vi "FP behavior P-Wall.vi"(1 "Behavior\nVelocity":dbl=20.0, 2 "Activate?":bool=TRUE, 3 "IR Sensors":T1(array[cluster])) -> (0 "P-Wall Array":dbl[](array[numeric]))   [LabVIEW 2014]
doc: "This vi creates a array based upon the value of the PBow IR sensor reading."
uses:
  <vilib>/addons/control/pid/pid.llb/PID (DBL).vi
  <vilib>/addons/control/pid/NI_PID_pid.lvlib
panel:
  out "HPort Setpoint":dbl=40.0 format="%#_13g"
  out "Half-Port\nSensor":string
  out "Port Setpoint":dbl=40.0 format="%#_13g"
  out "steer":dbl format="%.2f"
  out "Port Side Sensor":string
  out "Waveform Graph":cluster{dbl, dbl, dbl[]}(graph)
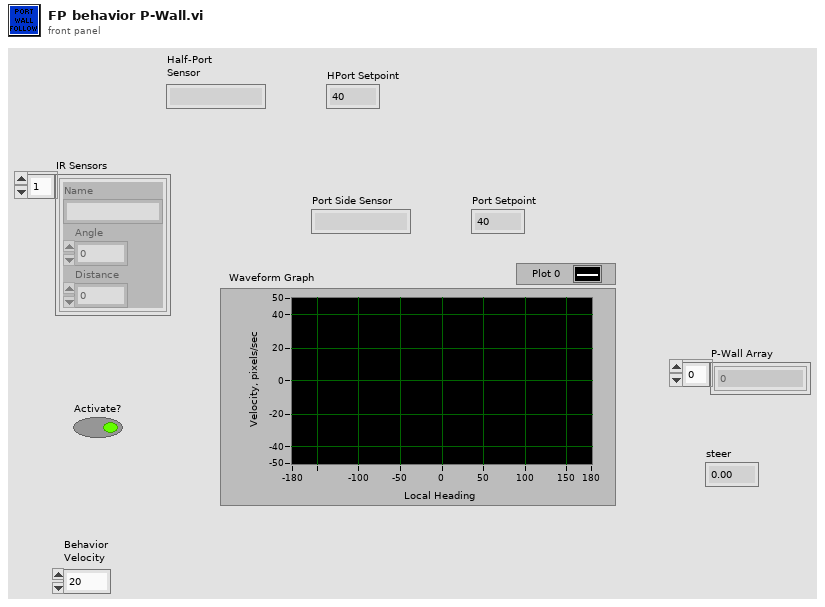
[diagram p1: front panel]
types:
  T1 = cluster{"Name":string, "Angle":dbl, "Distance":dbl}[]
  T2 = cluster{"proportional gain (Kc)":dbl, "integral time (Ti, min)":dbl, "derivative time (Td, min)":dbl}
  T3 = cluster{"Name":string, "Angle":dbl, "Distance":dbl}
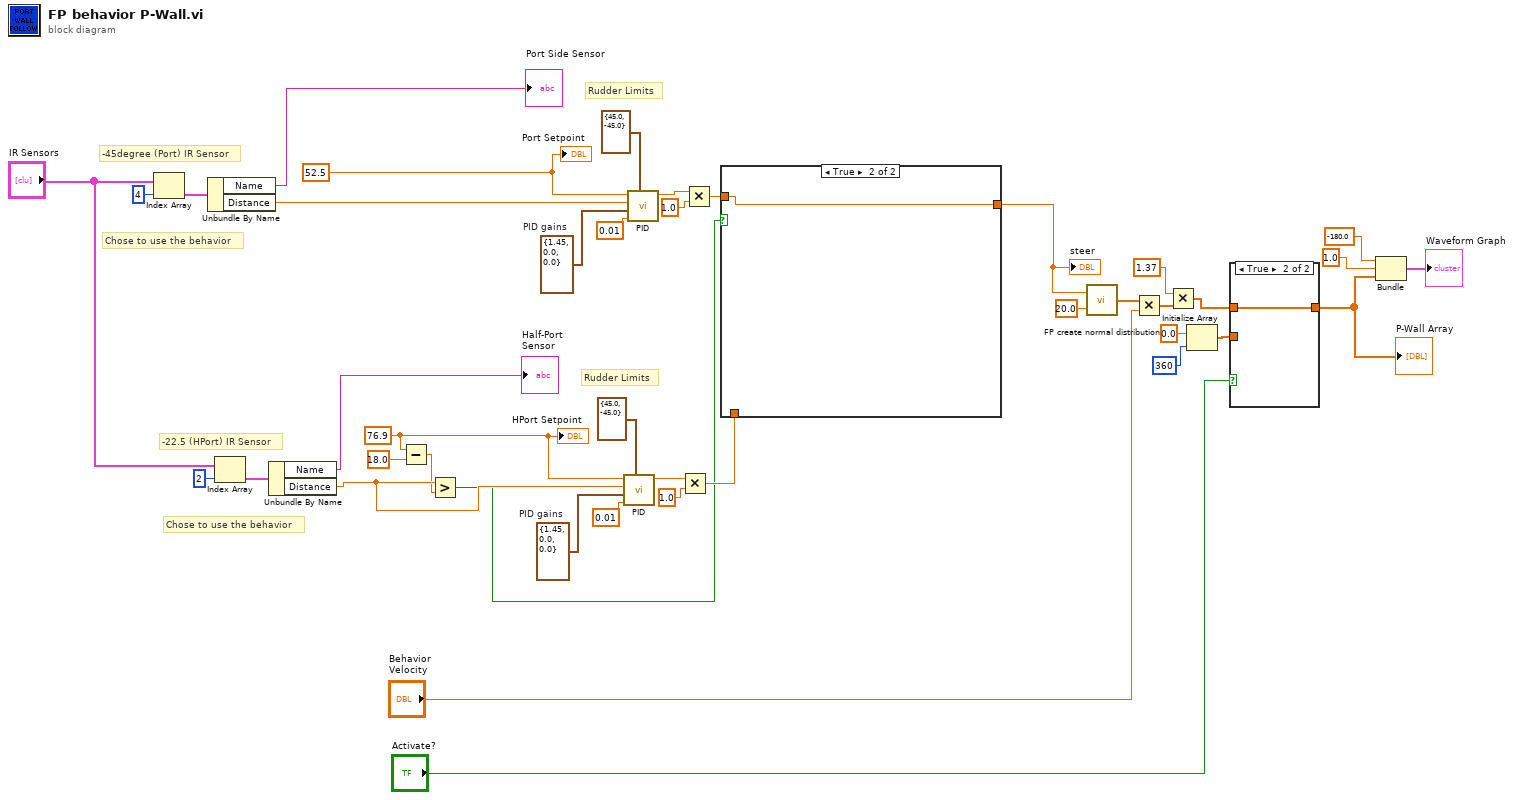
[diagram p0: block diagram]
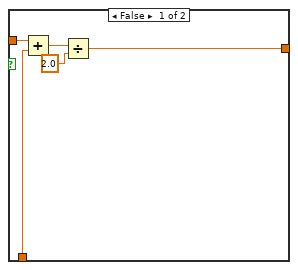
[diagram p2: hidden frame]
diagram:
  w3 = 76.9 ("Port Setpoint")
  w14 = 52.5 ("Port Setpoint")
  w16 = T2 {"proportional gain (Kc)"=1.45, "integral time (Ti, min)"=0.0, "derivative time (Td, min)"=0.0}  # PID gains
  w27 = T2 {"proportional gain (Kc)"=1.45, "integral time (Ti, min)"=0.0, "derivative time (Td, min)"=0.0}  # PID gains
  # "-22.5 (HPort) IR Sensor"
  # "-45degree (Port) IR Sensor"
  # "Rudder Limits"
  # "Chose to use the behavior"
  # "Rudder Limits"
  # "Chose to use the behavior"
  n1 = Index Array(array="IR Sensors", index=4) -> (element=w33:T3)
  n2 = Unbundle By Name(w33) -> ("Name"=→"Port Side Sensor":string, "Distance"=w6:dbl)
  n3 = Index Array(array="IR Sensors", index=2) -> (element=w22:T3)
  n4 = Unbundle By Name(w22) -> ("Name"=→"Half-Port\nSensor":string, "Distance"=w5:dbl)
  n5 = Subtract(x=w3, y=18.0) -> (x-y=w1:dbl)
  n6 = Greater?(x=w5, y=w1) -> (0:w4:bool)
  n7 = call-poly <vilib>:"PID.vi"("output range"=cluster{"output high":dbl, "output low":dbl} {"output high"=45.0, "output low"=-45.0}, "dt (s)"=0.01, "PID gains"=w16, "process variable"=w5, "setpoint"=w3) -> ("output"=w19:dbl)  [unwired: 5 in, 1 out]
  n8 = call-poly <vilib>:"PID.vi"("output range"=cluster{"output high":dbl, "output low":dbl} {"output high"=45.0, "output low"=-45.0}, "dt (s)"=0.01, "PID gains"=w27, "process variable"=w6, "setpoint"=w14) -> ("output"=w30:dbl)  [unwired: 5 in, 1 out]
  n9 = Multiply(x=w19, y=1.0) -> (x*y=w8:dbl)
  n10 = Multiply(x=w30, y=1.0) -> (x*y=w13:dbl)
  n11 = case shown="True" w4 {
    tunnel: w13 -> [w44 w47]
    tunnel: w8 -> [w43 _]
    tunnel: [w42 w47] -> w7
    frame False {
      n12 = Add(x=w44, y=w43) -> (x+y=w45:dbl)
      n13 = Divide(x=w45, y=2.0) -> (x/y=w42:dbl)
    }
    frame True {
    }
  }
  "steer" <- w7
  n14 = call "FP create normal distribution.vi"("std (Normal)"=20.0, "mean"=w7) -> ("ACT array"=w26:dbl[])
  n15 = Multiply(x=w26, y="Behavior\nVelocity") -> (x*y=w11:dbl[])
  n16 = Multiply(x=1.37, y=w11) -> (x*y=w9:dbl[])
  n17 = Initialize Array(0.0 ("element"), 360 ("dimension size")) -> (w36:dbl[])
  n18 = case shown="True" "Activate?" {
    tunnel: w36 -> [w48 _]
    tunnel: w9 -> [_ w49]
    tunnel: [w48 w49] -> w35
    frame False {
    }
    frame True {
    }
  }
  "P-Wall Array" <- w35
  n19 = Bundle(-180.0, 1.0, w35) -> (→"Waveform Graph":cluster{dbl, dbl, dbl[]})  [unwired: 1 in]
  "Port Setpoint" <- w14
  "HPort Setpoint" <- w3
